vi "Client2.vi"   [LabVIEW 2013]
uses:
  <vilib>/NXT/Block Support/NXT_ButtonSelector.ctl
  <vilib>/NXT/Block Support/NXT_MessageMailbox.ctl
  <vilib>/NXT/Subs/MotorOutput.ctl
  <vilib>/NXT/Dual Mode Library/Display/drawText.vi
  <vilib>/NXT/Dual Mode Library/BT/BlueTooth_Write_String.vi
types:
  T1 = typedef "LVHSConnector.ctl" = refnum<class "BrickReference.lvclass">
  T2 = typedef "NXT_ButtonSelector.ctl" = u16
  T3 = typedef "MotorOutput.ctl" = u8
  T4 = typedef "NXT_MessageMailbox.ctl" = u8
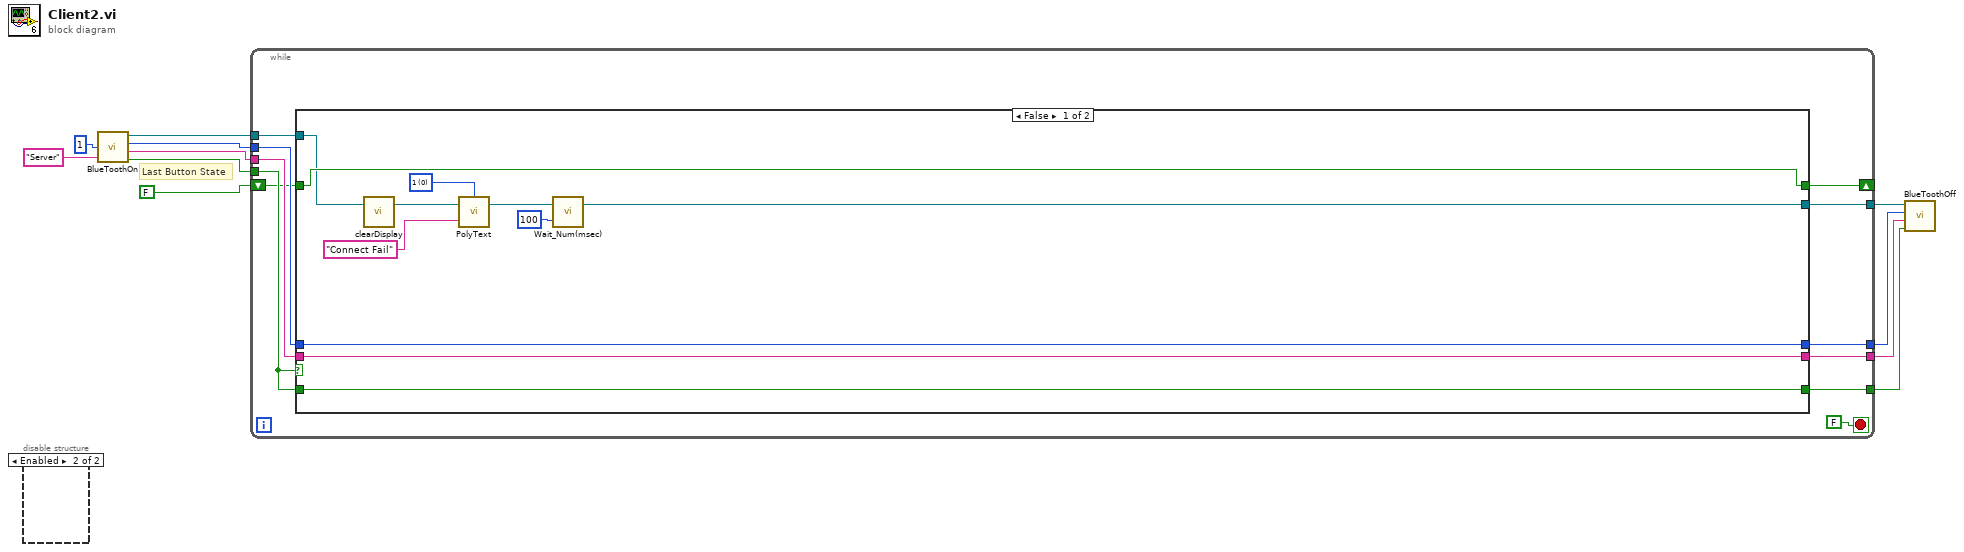
[diagram p0: block diagram]
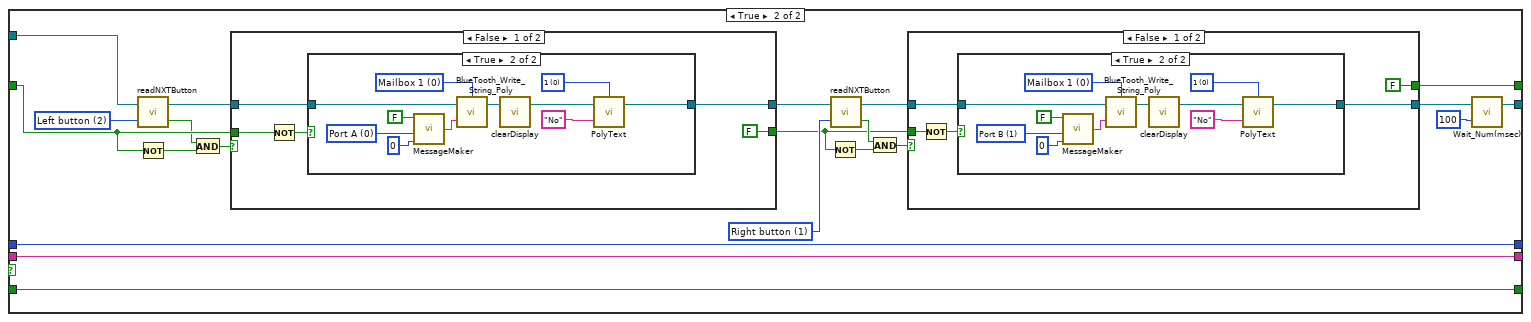
[diagram p2: hidden frame]
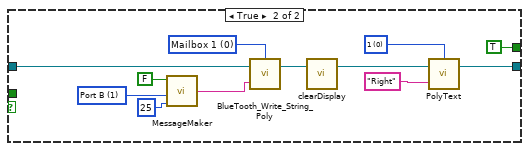
[diagram p4: hidden frame]
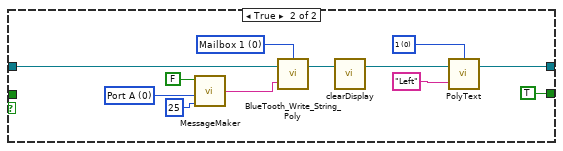
[diagram p6: hidden frame]
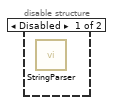
[diagram p7: hidden frame]
diagram:
  # "Last Button State"
  n1 = disable-structure shown="Enabled" {
    frame Disabled {
      n2 = call "StringParser.vi"() -> ()  [unwired: 1 in, 4 out]
    }
    frame Enabled {
    }
  }
  n3 = call "BlueToothOn.vi"("Connection"=u8 1, "Partner Name"="Server") -> ("NXT/EV3 2"=w9:T1, "Connection"=w8:u8, "Partner Name"=w7:string, "Success"=w6:bool)  [unwired: 1 in]
  n4 = while {
    tunnel: w9 -> [w22]
    tunnel: w8 -> [w21]
    tunnel: w7 -> [w20]
    tunnel: w6 -> [w19]
    tunnel: [w18] -> w5
    tunnel: [w17] -> w4
    tunnel: [w16] -> w3
    tunnel: [w15] -> w2
    shift-right: [w12] -> _
    shift-left: FALSE -> [w13]
    stop <- FALSE stop-if-true
    n5 = case shown="False" w19 {
      tunnel: w22 -> [w28 w50]
      tunnel: w21 -> [w33 w52]
      tunnel: w20 -> [w32 w53]
      tunnel: [w24 w35] -> w15
      tunnel: [w33 w52] -> w16
      tunnel: [w32 w53] -> w17
      tunnel: w19 -> [w31 w54]
      tunnel: [w31 w54] -> w18
      tunnel: w13 -> [w30 w47]
      tunnel: [w30 w34] -> w12
      frame False {
        w27 = i16 0 items=["1", "2", "3", "4", "5", "6", "7", "8", "9", "10", "11", "12"] ("Line")
        n6 = call <vilib>:"clearDisplay.vi"("NXT/EV3"=w28) -> ("NXT/EV3"=w29:T1)  [unwired: 3 in]
        n7 = call-poly <vilib>:"PolyText.vi"("Text"="Connect Fail", "NXT/EV3"=w29, "Line"=w27) -> ("NXT/EV3"=w25:T1)  [unwired: 1 in]
        n8 = call <vilib>:"Wait_Num(msec).vi"("Time (100 msec)"=u32 100, "NXT/EV3"=w25) -> ("NXT/EV3"=w24:T1)  [unwired: 2 in]
      }
      frame True {
        w43 = T2 1 items=["Enter button"=3, "Left button"=2, "Right button"=1, "Up Button"=4, "Down Button"=5] ("Button (Enter button)")
        w51 = T2 2 items=["Enter button"=3, "Left button"=2, "Right button"=1, "Up Button"=4, "Down Button"=5] ("Button (Enter button)")
        n9 = call <vilib>:"readNXTButton.vi"("Button (Enter button)"=w51, "NXT/EV3"=w50) -> ("Yes/No"=w46:bool, "NXT/EV3"=w49:T1)  [unwired: 1 in]
        n10 = Not(x=w47) -> (.not. x?=w48:bool)
        n11 = And(x=w46, y=w48) -> (x .and. y?=w45:bool)
        n12 = case shown="False" w45 {
          tunnel: [w86 w103] -> w39
          tunnel: w49 -> [w87 w107]
          tunnel: w47 -> [w85 _]
          tunnel: [FALSE TRUE] -> w36
          frame False {
            n13 = Not(x=w85) -> (.not. x?=w84:bool)
            n14 = case shown="True" w84 {
              tunnel: w87 -> [w89 w95]
              tunnel: [w89 w92] -> w86
              frame False {
              }
              frame True {
                w90 = i16 0 items=["1", "2", "3", "4", "5", "6", "7", "8", "9", "10", "11", "12"] ("Line")
                w99 = T3 0 items=["Port A"=0, "Port B"=1, "Port C"=2, "Ports A & B"=4, "Ports A & C"=5, "Ports B & C"=6, "All Ports"=3] ("Output Port (All Ports)")
                w97 = T4 0 items=["Mailbox 1", "Mailbox 2", "Mailbox 3", "Mailbox 4", "Mailbox 5", "Mailbox 6", "Mailbox 7", "Mailbox 8", "Mailbox 9", "Mailbox 10"] ("Mailbox")
                n15 = call "MessageMaker.vi"("Power"=0, "Output Port (All Ports)"=w99, "R/W (T=R/F=W)"=FALSE) -> ("Message"=w96:string)  [unwired: 1 in]
                n16 = call-poly <vilib>:"BlueTooth_Write_String_Poly.vi"("Message"=w96, "NXT/EV3"=w95, "Mailbox"=w97) -> ("NXT/EV3"=w94:T1)  [unwired: 1 in]
                n17 = call <vilib>:"clearDisplay.vi"("NXT/EV3"=w94) -> ("NXT/EV3"=w93:T1)  [unwired: 3 in]
                n18 = call-poly <vilib>:"PolyText.vi"("Text"="No", "NXT/EV3"=w93, "Line"=w90) -> ("NXT/EV3"=w92:T1)  [unwired: 1 in]
              }
            }
          }
          frame True {
            w101 = i16 0 items=["1", "2", "3", "4", "5", "6", "7", "8", "9", "10", "11", "12"] ("Line")
            w109 = T3 0 items=["Port A"=0, "Port B"=1, "Port C"=2, "Ports A & B"=4, "Ports A & C"=5, "Ports B & C"=6, "All Ports"=3] ("Output Port (All Ports)")
            w111 = T4 0 items=["Mailbox 1", "Mailbox 2", "Mailbox 3", "Mailbox 4", "Mailbox 5", "Mailbox 6", "Mailbox 7", "Mailbox 8", "Mailbox 9", "Mailbox 10"] ("Mailbox")
            n19 = call "MessageMaker.vi"("Power"=25, "Output Port (All Ports)"=w109, "R/W (T=R/F=W)"=FALSE) -> ("Message"=w112:string)  [unwired: 1 in]
            n20 = call-poly <vilib>:"BlueTooth_Write_String_Poly.vi"("Message"=w112, "NXT/EV3"=w107, "Mailbox"=w111) -> ("NXT/EV3"=w104:T1)  [unwired: 1 in]
            n21 = call <vilib>:"clearDisplay.vi"("NXT/EV3"=w104) -> ("NXT/EV3"=w105:T1)  [unwired: 3 in]
            n22 = call-poly <vilib>:"PolyText.vi"("Text"="Left", "NXT/EV3"=w105, "Line"=w101) -> ("NXT/EV3"=w103:T1)  [unwired: 1 in]
          }
        }
        n23 = Not(x=w36) -> (.not. x?=w42:bool)
        n24 = call <vilib>:"readNXTButton.vi"("Button (Enter button)"=w43, "NXT/EV3"=w39) -> ("Yes/No"=w41:bool, "NXT/EV3"=w38:T1)  [unwired: 1 in]
        n25 = And(x=w41, y=w42) -> (x .and. y?=w40:bool)
        n26 = case shown="False" w40 {
          tunnel: [w57 w74] -> w37
          tunnel: w38 -> [w58 w78]
          tunnel: w36 -> [w56 _]
          tunnel: [FALSE TRUE] -> w34
          frame False {
            n27 = Not(x=w56) -> (.not. x?=w55:bool)
            n28 = case shown="True" w55 {
              tunnel: w58 -> [w60 w66]
              tunnel: [w60 w63] -> w57
              frame False {
              }
              frame True {
                w61 = i16 0 items=["1", "2", "3", "4", "5", "6", "7", "8", "9", "10", "11", "12"] ("Line")
                w70 = T3 1 items=["Port A"=0, "Port B"=1, "Port C"=2, "Ports A & B"=4, "Ports A & C"=5, "Ports B & C"=6, "All Ports"=3] ("Output Port (All Ports)")
                w68 = T4 0 items=["Mailbox 1", "Mailbox 2", "Mailbox 3", "Mailbox 4", "Mailbox 5", "Mailbox 6", "Mailbox 7", "Mailbox 8", "Mailbox 9", "Mailbox 10"] ("Mailbox")
                n29 = call "MessageMaker.vi"("Power"=0, "Output Port (All Ports)"=w70, "R/W (T=R/F=W)"=FALSE) -> ("Message"=w67:string)  [unwired: 1 in]
                n30 = call-poly <vilib>:"BlueTooth_Write_String_Poly.vi"("Message"=w67, "NXT/EV3"=w66, "Mailbox"=w68) -> ("NXT/EV3"=w65:T1)  [unwired: 1 in]
                n31 = call <vilib>:"clearDisplay.vi"("NXT/EV3"=w65) -> ("NXT/EV3"=w64:T1)  [unwired: 3 in]
                n32 = call-poly <vilib>:"PolyText.vi"("Text"="No", "NXT/EV3"=w64, "Line"=w61) -> ("NXT/EV3"=w63:T1)  [unwired: 1 in]
              }
            }
          }
          frame True {
            w72 = i16 0 items=["1", "2", "3", "4", "5", "6", "7", "8", "9", "10", "11", "12"] ("Line")
            w80 = T3 1 items=["Port A"=0, "Port B"=1, "Port C"=2, "Ports A & B"=4, "Ports A & C"=5, "Ports B & C"=6, "All Ports"=3] ("Output Port (All Ports)")
            w82 = T4 0 items=["Mailbox 1", "Mailbox 2", "Mailbox 3", "Mailbox 4", "Mailbox 5", "Mailbox 6", "Mailbox 7", "Mailbox 8", "Mailbox 9", "Mailbox 10"] ("Mailbox")
            n33 = call "MessageMaker.vi"("Power"=25, "Output Port (All Ports)"=w80, "R/W (T=R/F=W)"=FALSE) -> ("Message"=w83:string)  [unwired: 1 in]
            n34 = call-poly <vilib>:"BlueTooth_Write_String_Poly.vi"("Message"=w83, "NXT/EV3"=w78, "Mailbox"=w82) -> ("NXT/EV3"=w75:T1)  [unwired: 1 in]
            n35 = call <vilib>:"clearDisplay.vi"("NXT/EV3"=w75) -> ("NXT/EV3"=w76:T1)  [unwired: 3 in]
            n36 = call-poly <vilib>:"PolyText.vi"("Text"="Right", "NXT/EV3"=w76, "Line"=w72) -> ("NXT/EV3"=w74:T1)  [unwired: 1 in]
          }
        }
        n37 = call <vilib>:"Wait_Num(msec).vi"("Time (100 msec)"=u32 100, "NXT/EV3"=w37) -> ("NXT/EV3"=w35:T1)  [unwired: 2 in]
      }
    }
  }
  n38 = call "BlueToothOff.vi"("Connected"=w5, "Partner Name"=w4, "Connection"=w3, "NXT/EV3"=w2) -> ()  [unwired: 1 in, 3 out]
